vi "PowerSlideDriveMotors.vi"(4 "Reduction":dbl, 6 "TurnThreshold":dbl, 8 "error in (no error)":errorcluster, 9 "RightSpeed":dbl, 10 "LeftSpeed":dbl, 11 "RobotDriveDevRef 2":T1={"DevStatus"={"status"=FALSE, "code"=0, "source"=""}, "Motors[]"=[], "Square Inputs"=FALSE, "Max Output"=1.0}) -> (0 "error out":errorcluster, 2 "Motor Values":dbl[](array[numeric]), 3 "RobotDriveDevRef":T1={"DevStatus"={"status"=FALSE, "code"=0, "source"=""}, "Motors[]"=[], "Square Inputs"=FALSE, "Max Output"=1.0})   [LabVIEW 2014, in "PowerSlide.lvlib"]
uses:
  PowerSlide.lvlib
  <vilib>/Rock Robotics/WPI/RobotDrive/WPI_RobotDriveDevRef.ctl
  <vilib>/Rock Robotics/WPI/MotorControl/WPI_MotorControlDeviceRef.ctl
  <vilib>/Rock Robotics/WPI/MotorControl/WPI_MotorControlType.ctl
  <vilib>/Rock Robotics/SystemInterfaces/Typedef/FPGA_TypedefDigitalModule.ctl
  <vilib>/Rock Robotics/SystemInterfaces/DIO/FPGA_DIOPWMChannel.ctl
  <vilib>/Rock Robotics/WPI/PWM/WPI_PWMDeadband.ctl
  <vilib>/Rock Robotics/WPI/CAN/Jaguar/SubVIs/WPI_CANJaguar_ControlMode.ctl
  <vilib>/Rock Robotics/WPI/CAN/TalonSRX/WPI_CANTalonSRX_APIControlMode.ctl
  <vilib>/Rock Robotics/WPI/PWM/WPI_PWMTransform_ConPane.ctl
  <vilib>/Rock Robotics/WPI/RobotDrive/WPI_RobotDriveMotorSelectorEnum.ctl
  <vilib>/Rock Robotics/WPI/RobotDrive/WPI_RobotDriveSafetyCheck.vi
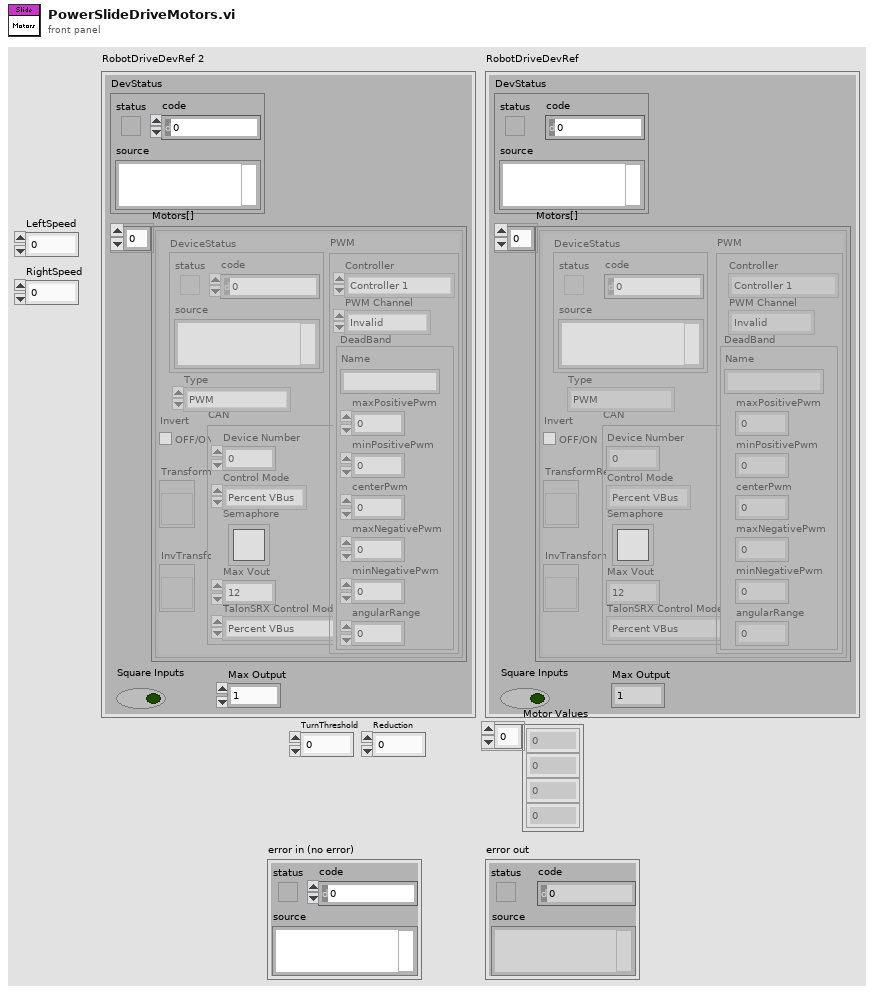
[diagram p1: front panel]
types:
  T1 = typedef "WPI_RobotDriveDevRef.ctl" = cluster{"DevStatus":errorcluster, "Motors[]":T2[], "Square Inputs":bool, "Max Output":dbl}
  T2 = typedef "WPI_MotorControlDeviceRef.ctl" = cluster{"DeviceStatus":errorcluster, "Type":T3, "PWM":cluster{"Controller":T4, "PWM Channel":T5, "DeadBand":T6}, "CAN":cluster{"Device Number":u8, "Control Mode":T7, "Semaphore":T8, "Max Vout":dbl, "TalonSRX Control Mode":T9}, "Invert":bool, "TransformRef":T10, "InvTransformRef":T10}
  T3 = typedef "WPI_MotorControlType.ctl" = enum16{"PWM", "CAN", "CANTalonSRX"}
  T4 = typedef "FPGA_TypedefDigitalModule.ctl" = enum16{"Controller 1"}
  T5 = typedef "FPGA_DIOPWMChannel.ctl" = enum8{"PWM 0", "PWM 1", "PWM 2", "PWM 3", "PWM 4", "PWM 5", "PWM 6", "PWM 7", "PWM 8", "PWM 9", "PWM MXP 0", "PWM MXP 1", "PWM MXP 2", "PWM MXP 3", "PWM MXP 4", "PWM MXP 5", "PWM MXP 6", "PWM MXP 7", "PWM MXP 8", "PWM MXP 9", "Invalid"}
  T6 = typedef "WPI_PWMDeadband.ctl" = cluster{"Name":string, "maxPositivePwm":i32, "minPositivePwm":i32, "centerPwm":i32, "maxNegativePwm":i32, "minNegativePwm":i32, "angularRange":u16}
  T7 = typedef "WPI_CANJaguar_ControlMode.ctl" = enum8{"Percent VBus", "Current", "Speed", "Position", "Voltage"}
  T8 = typedef "Semaphore RefNum" = refnum<k1>
  T9 = typedef "WPI_CANTalonSRX_APIControlMode.ctl" = enum8{"Percent VBus", "Speed", "Position", "Slave", "Unchanged / Invalid"}
  T10 = typedef "WPI_PWMTransform_ConPane.ctl" = refnum<vi>
  T11 = typedef "WPI_RobotDriveMotorSelectorEnum.ctl" = enum16{"Rear Left Motor", "Rear Right Motor", "Front Left Motor", "Front Right Motor"}
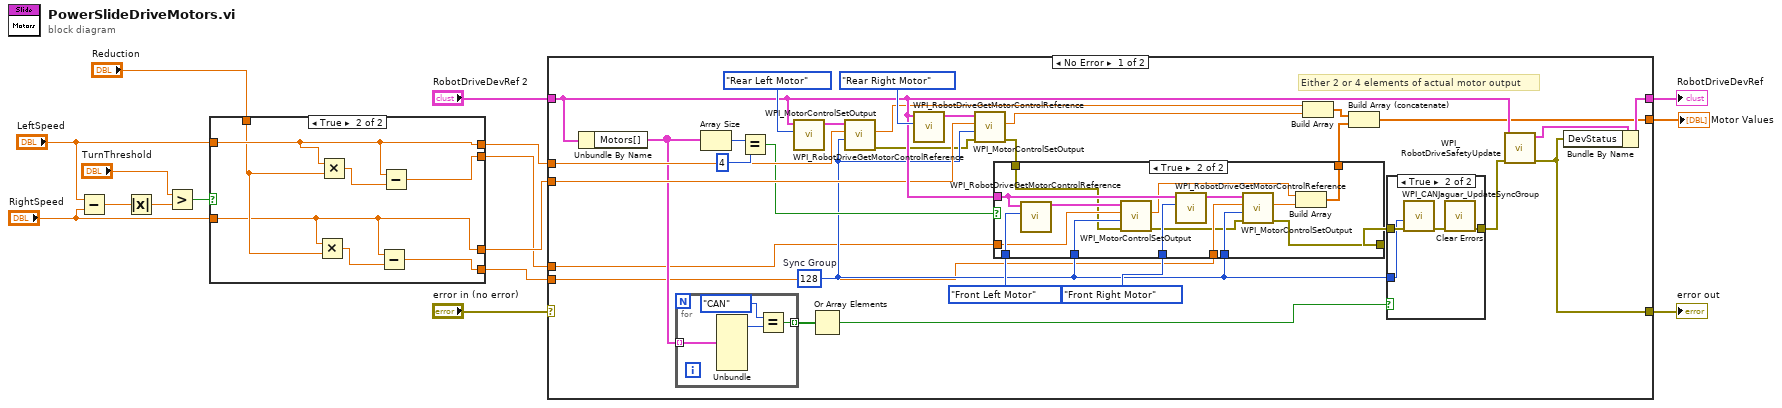
[diagram p0: block diagram]
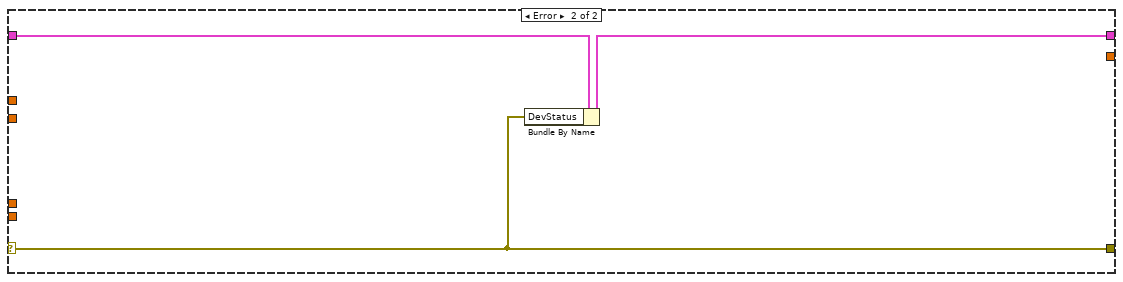
[diagram p5: hidden frame]
diagram:
  n1 = Subtract(x="LeftSpeed", y="RightSpeed") -> (x-y=w11:dbl)
  n2 = Absolute Value(x=w11) -> (abs(x)=w10:dbl)
  n3 = Greater?(x="TurnThreshold", y=w10) -> (0:w8:bool)
  n4 = case shown="True" w8 {
    tunnel: [w18 w25] -> w7
    tunnel: "LeftSpeed" -> [w18 w25]
    tunnel: "RightSpeed" -> [w17 w19]
    tunnel: [w17 w19] -> w4
    tunnel: [w18 w23] -> w3
    tunnel: [w17 w21] -> w2
    tunnel: "Reduction" -> [_ w20]
    frame False {
    }
    frame True {
      n5 = Multiply(x=w19, y=w20) -> (x*y=w22:dbl)
      n6 = Multiply(x=w25, y=w20) -> (x*y=w24:dbl)
      n7 = Subtract(x=w19, y=w22) -> (x-y=w21:dbl)
      n8 = Subtract(x=w25, y=w24) -> (x-y=w23:dbl)
    }
  }
  n9 = case shown="No Error" "error in (no error)" {
    selector: "error in (no error)" -> [_ w82]
    tunnel: "RobotDriveDevRef 2" -> [w47 w83]
    tunnel: [w44 w81] -> w15
    tunnel: w7 -> [w42 _]
    tunnel: w4 -> [w43 _]
    tunnel: [w45 w82] -> w13
    tunnel: [w28 _] -> w12
    tunnel: w3 -> [w27 _]
    tunnel: w2 -> [w26 _]
    frame No Error {
      w40 = u8 128  # Sync Group
      # "Either 2 or 4 elements of actual motor output"
      n10 = Unbundle By Name(w47) -> ("Motors[]"=w39:T2[])
      n11 = for {
        tunnel: w39 -> [w59] mode=indexing
        tunnel: [w56] -> w38 mode=indexing
        n12 = Unbundle(w59) -> ("Type"=w58:T3)  [unwired: 6 out]
        n13 = Equal?(x=enum16{"PWM", "CAN"}."CAN" ("Type"), y=w58) -> (x = y?=w56:bool)
      }
      n14 = Array Size(array=w39) -> (size(s)=w55:i32)
      n15 = Equal?(x=w55, y=4) -> (x = y?=w41:bool)
      n16 = call <vilib>:"WPI_RobotDriveGetMotorControlReference.vi"("MotorIndex"=WPI_RobotDriveMotorSelectorEnum."Rear Left Motor", "RobotDriveDevRef"=w47) -> ("MotorControlDeviceRef"=w52:T2)  [unwired: 9 out]
      n17 = Or Array Elements(Boolean array=w38) -> (logical OR=w37:bool)
      n18 = call <vilib>:"WPI_MotorControlSetOutput.vi"("Sync Group / Parameter Slot"=w40, "Output"=w42, "MotorControlDevRef"=w52) -> ("error out"=w36:errorcluster, "Motor Output"=w32:dbl)  [unwired: 2 in, 5 out]
      n19 = call <vilib>:"WPI_RobotDriveGetMotorControlReference.vi"("MotorIndex"=WPI_RobotDriveMotorSelectorEnum."Rear Right Motor", "RobotDriveDevRef"=w47) -> ("MotorControlDeviceRef"=w53:T2)  [unwired: 9 out]
      n20 = call <vilib>:"WPI_MotorControlSetOutput.vi"("error in (no error)"=w36, "Sync Group / Parameter Slot"=w40, "Output"=w43, "MotorControlDevRef"=w53) -> ("error out"=w34:errorcluster, "Motor Output"=w31:dbl)  [unwired: 1 in, 5 out]
      n21 = case shown="True" w41 {
        tunnel: WPI_RobotDriveMotorSelectorEnum."Front Left Motor" ("MotorIndex") -> [_ w80]
        tunnel: WPI_RobotDriveMotorSelectorEnum."Front Right Motor" ("MotorIndex") -> [_ w79]
        tunnel: w47 -> [_ w78]
        tunnel: w40 -> [_ w77]
        tunnel: w26 -> [_ w76]
        tunnel: w27 -> [_ w75]
        tunnel: [w65 w71] -> w35
        tunnel: w40 -> [_ w72]
        tunnel: w34 -> [w65 w69]
        tunnel: [_ w66] -> w30
        frame False {
        }
        frame True {
          n22 = call <vilib>:"WPI_RobotDriveGetMotorControlReference.vi"("MotorIndex"=w80, "RobotDriveDevRef"=w78) -> ("MotorControlDeviceRef"=w73:T2)  [unwired: 9 out]
          n23 = call <vilib>:"WPI_MotorControlSetOutput.vi"("error in (no error)"=w69, "Sync Group / Parameter Slot"=w72, "Output"=w75, "MotorControlDevRef"=w73) -> ("error out"=w70:errorcluster, "Motor Output"=w67:dbl)  [unwired: 1 in, 5 out]
          n24 = call <vilib>:"WPI_RobotDriveGetMotorControlReference.vi"("MotorIndex"=w79, "RobotDriveDevRef"=w78) -> ("MotorControlDeviceRef"=w74:T2)  [unwired: 9 out]
          n25 = call <vilib>:"WPI_MotorControlSetOutput.vi"("error in (no error)"=w70, "Sync Group / Parameter Slot"=w77, "Output"=w76, "MotorControlDevRef"=w74) -> ("error out"=w71:errorcluster, "Motor Output"=w68:dbl)  [unwired: 1 in, 5 out]
          n26 = Build Array(w67, w68) -> (w66:dbl[])
        }
      }
      n27 = Build Array(w32, w31) -> (w29:dbl[])
      n28 = Build Array (concatenate)(w29, w30) -> (w28:dbl[])
      n29 = case shown="True" w37 {
        tunnel: w35 -> [w60 w63]
        tunnel: w40 -> [_ w62]
        tunnel: [w60 w61] -> w33
        frame False {
        }
        frame True {
          n30 = call <vilib>:"WPI_CANJaguar_UpdateSyncGroup.vi"("error in (no error)"=w63, "Sync Group"=w62) -> ("error out"=w64:errorcluster)  [unwired: 9 out]
          n31 = call <vilib>:"Clear Errors.vi"("error in (no error)"=w64) -> ("error out"=w61:errorcluster)  [unwired: 1 in, 5 out]
        }
      }
      n32 = call <vilib>:"WPI_RobotDriveSafetyUpdate.vi"("error in (no error)"=w33, "RobotDriveDevRef"=w47) -> ("error out"=w45:errorcluster, "RobotDriveDevRef"=w46:T1)  [unwired: 8 out]
      n33 = Bundle By Name(cluster=w46, "DevStatus"=w45) -> (w44:T1)
    }
    frame Error {
      n34 = Bundle By Name(cluster=w83, "DevStatus"=w82) -> (w81:T1)
    }
  }
  "RobotDriveDevRef" <- w15
  "error out" <- w13
  "Motor Values" <- w12
